vi "Get Trigger Model LAN Overrun Status.vi"(8 "error in (no error)":errorcluster, 10 "LAN Event Number (1)":i32=1 format="%#.6g", 11 "VISA resource name":refnum<visa-resource-name>) -> (0 "error out":errorcluster, 2 "Overrun Status":bool, 3 "VISA resource name out":refnum<visa-resource-name>)   [LabVIEW 2021, in "Keithley 2450.lvlib"]
doc: "Indicates the overrun status of the event detector."
uses:
  <instrlib>/Keithley 2450/Keithley 2450.lvlib
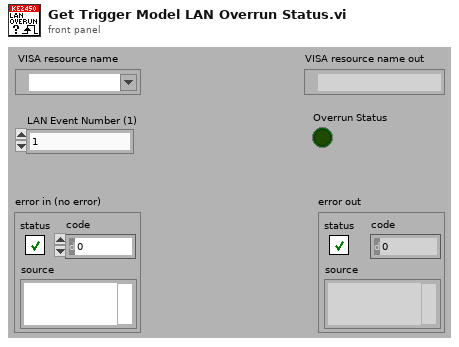
[diagram p1: front panel]
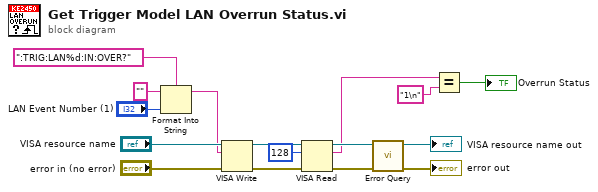
[diagram p0: block diagram]
diagram:
  n1 = Format Into String(format string=":TRIG:LAN%d:IN:OVER?", initial string="", "LAN Event Number (1)") -> (resulting string=w4:string)  [unwired: 1 in, 1 out]
  n2 = VISA Write(VISA resource name="VISA resource name", write buffer=w4, error in (no error)="error in (no error)") -> (VISA resource name out=w10:refnum<visa-resource-name>, error out=w12:errorcluster)  [unwired: 1 out]
  n3 = VISA Read(VISA resource name=w10, byte count=u32 128, error in (no error)=w12) -> (VISA resource name out=w9:refnum<visa-resource-name>, read buffer=w1:string, error out=w11:errorcluster)  [unwired: 1 out]
  n4 = call <instrlib>:"Error Query.vi"("error in (no error)"=w11, "VISA resource name"=w9) -> ("error out"=→"error out":errorcluster, "VISA resource name out"=→"VISA resource name out":refnum<visa-resource-name>)  [unwired: 8 out]
  n5 = Equal?(x=w1, y="1\n") -> (x = y?=→"Overrun Status":bool)
